vi "Set Power Cell Visibility.vi"(9 "Show":bool, 10 "Ball Slot":i32, 11 "Knob in":refnum<vi>) -> (3 "Knob out":refnum<vi>)   [LabVIEW 2019]
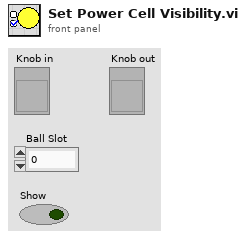
[diagram p1: front panel]
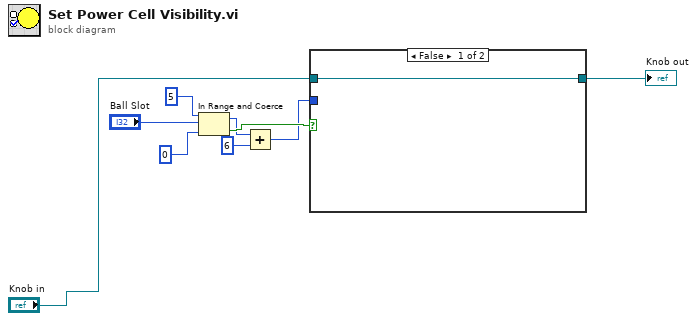
[diagram p0: block diagram]
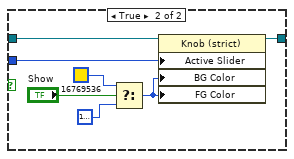
[diagram p2: hidden frame]
diagram:
  n1 = In Range and Coerce(upper limit=5, x="Ball Slot", lower limit=0) -> (coerced(x)=w5:i32, In Range?=w9:bool)
  n2 = Add(x=w5, y=6) -> (x+y=w7:i32)
  n3 = case shown="False" w9 {
    tunnel: "Knob in" -> [w10 w17]
    tunnel: w7 -> [_ w16]
    tunnel: [w10 w11] -> w8
    frame False {
    }
    frame True {
      n4 = Select(t=u32 16769536 ("Housing Colors:FG Color"), s="Show", f=u32 16777216 ("Housing Colors:FG Color")) -> (s? t:f=w12:u32)
      n5 = property on="Property Node" class="Knob (strict)"(reference=w17, "Active Slider"=w16, "BG Color"=w12, "FG Color"=w12) -> (reference out=w11:refnum<vi>)  [unwired: 1 in, 1 out]
    }
  }
  "Knob out" <- w8
